vi "Send Stop.vi"(8 "error in (no error)":errorcluster, 11 "Message Queue":refnum<queue>) -> (0 "error out":errorcluster)   [LabVIEW 2024, in "Zero Timeout Message Handler.lvlib" / "Stop Msg.lvclass"]
uses:
  Stop Msg.lvclass
  ~Message/~Message.lvclass
  Stop Msg.lvclass/Stop Msg.ctl
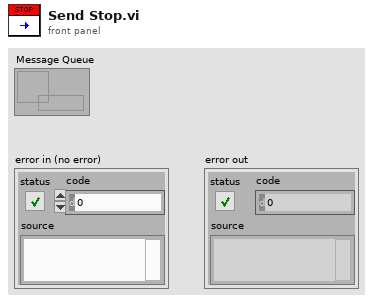
[diagram p1: front panel]
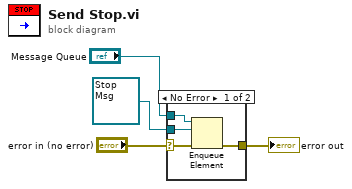
[diagram p0: block diagram]
diagram:
  n1 = case shown="No Error" "error in (no error)" {
    selector: "error in (no error)" -> [w5 w9]
    tunnel: "Message Queue" -> [w8 _]
    tunnel: refnum<class "Stop Msg.lvclass"> refnum ("Zero Timeout Message Handler.lvlib:Stop Msg.lvclass") -> [w7 _]
    tunnel: [w6 w9] -> w2
    frame No Error {
      n2 = Enqueue Element(queue=w8, element=w7, error in (no error)=w5) -> (error out=w6:errorcluster)  [unwired: 1 in, 2 out]
    }
    frame Error {
    }
  }
  "error out" <- w2
